vi "Create Server.vi"(5 "Server in":refnum<class "Server.lvclass">, 6 "Max QoS Supported (QoS = 2)":T1=enum."2 (Exactly Once)", 8 "error in (no error)":errorcluster, 11 "Connection Configuration":refnum<class "Connection.lvclass">) -> (0 "error out":errorcluster, 3 "Server":refnum<class "Server.lvclass">)   [LabVIEW 2013, in "MQTT Server.lvlib" / "Server.lvclass"]
uses:
  Server.lvclass
  <vilib>/LabVIEW Open Source Project/MQTT Control Packets/Control Packets/ControlPacket/QualityOfService -- enum.ctl
  <vilib>/LabVIEW Open Source Project/MQTT Connection/MQTT_Connection/Connection/Connection.lvclass
  <vilib>/LabVIEW Open Source Project/MQTT Connection/MQTT_Base/Base Class/MQTT_Base.lvclass/MQTT_Base.ctl
  Server.lvclass/Server.ctl
  <vilib>/LabVIEW Open Source Project/MQTT Connection/MQTT_Base/Base Class/MQTT_Base.lvclass
  <vilib>/LabVIEW Open Source Project/MQTT Control Packets/Control Packets/ControlPacket/ControlPacket.lvclass
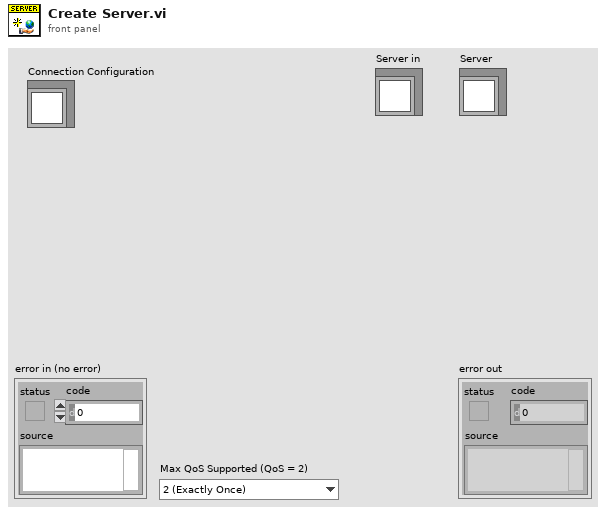
[diagram p1: front panel]
types:
  T1 = typedef "MQTT_Control_Packets.lvlib/ControlPacket.lvclass/QualityOfService -- enum.ctl" = enum16{"0 (At Most Once)", "1 (At Least Once)", "2 (Exactly Once)"}
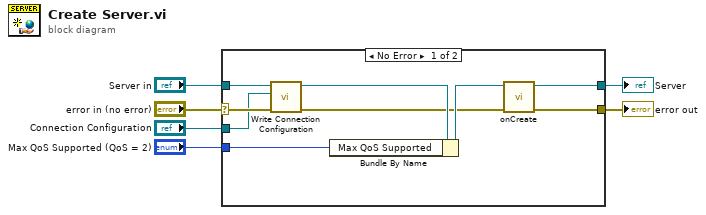
[diagram p0: block diagram]
diagram:
  n1 = case shown="No Error" "error in (no error)" {
    selector: "error in (no error)" -> [w9 w17]
    tunnel: [w15 w17] -> w5
    tunnel: [w13 w16] -> w3
    tunnel: "Server in" -> [w11 w16]
    tunnel: "Max QoS Supported (QoS = 2)" -> [w14 _]
    tunnel: "Connection Configuration" -> [w7 _]
    frame No Error {
      n2 = call <vilib>:"Write Connection Configuration.vi"("error in (no error)"=w9, "Connection Configuration"=w7, "MQTT_Base in"=w11) -> ("error out"=w8:errorcluster, "MQTT_Base out"=w10:refnum<class "Server.lvclass">)  [unwired: 7 in]
      n3 = Bundle By Name(cluster=w10, "Max QoS Supported"=w14) -> (w12:refnum<class "Server.lvclass">)
      n4 = call-dynamic "onCreate.vi"("error in (no error)"=w8, "Server in"=w12) -> ("error out"=w15:errorcluster, "Server out"=w13:refnum<class "Server.lvclass">)  [unwired: 8 in]
    }
    frame Error {
    }
  }
  "error out" <- w5
  "Server" <- w3
